vi "WaveformSimulatorFINAL.vi"(9 "Waveform Parameters":T1={"Frequency"=50.0, "Amplitude"=5.0, "Shape"=enum."Sine"}, 10 "Digitizing Parameters":T2={"Number of Samples"=100, "Sampling Frequency"=1000.0}) -> (2 "Waveform Output":cluster{"Time":dbl[], "Displacement":dbl[]}={"Time"=[0.0, 0.001, 0.002, 0.003, 0.004, 0.005, 0.006, 0.007, 0.008, 0.009000000000000001, 0.01, 0.011, 0.012, 0.013000000000000001, 0.014, 0.015, 0.016, 0.017, 0.018000000000000002, 0.019, 0.02, 0.021, 0.022, 0.023, 0.024, 0.025, 0.026000000000000002, 0.027, 0.028, 0.029, 0.03, 0.031, 0.032, 0.033, 0.034, 0.035, 0.036000000000000004, 0.037, 0.038, 0.039, 0.04, 0.041, 0.042, 0.043000000000000003, 0.044, 0.045, 0.046, 0.047, 0.048, 0.049, 0.05, 0.051000000000000004, 0.052000000000000005, 0.053, 0.054, 0.055, 0.056, 0.057, 0.058, 0.059000000000000004, 0.06, 0.061, 0.062, 0.063, 0.064, 0.065, 0.066, 0.067, 0.068, 0.069, 0.07, 0.07100000000000001, 0.07200000000000001, 0.073, 0.074, 0.075, 0.076, 0.077, 0.078, 0.079, 0.08, 0.081, 0.082, 0.083, 0.084, 0.085, 0.08600000000000001, 0.08700000000000001, 0.088, 0.089, 0.09, 0.091, 0.092, 0.093, 0.094, 0.095, 0.096, 0.097, 0.098, 0.099], "Displacement"=[0.0, 1.545084971874737, 2.938926261462366, 4.045084971874737, 4.755282581475767, 5.0, 4.755282581475767, 4.045084971874737, 2.9389262614623664, 1.5450849718747355, 6.123233995736766e-16, -1.5450849718747364, -2.938926261462367, -4.04508497187474, -4.755282581475767, -5.0, -4.755282581475768, -4.045084971874735, -2.938926261462363, -1.5450849718747381, -1.2246467991473533e-15, 1.54508497187474, 2.9389262614623646, 4.045084971874736, 4.755282581475769, 5.0, 4.7552825814757655, 4.045084971874738, 2.938926261462367, 1.545084971874739, 1.8369701987210296e-15, -1.5450849718747353, -2.938926261462364, -4.045084971874741, -4.75528258147577, -5.0, -4.755282581475766, -4.045084971874738, -2.9389262614623672, -1.5450849718747395, -2.4492935982947065e-15, 1.545084971874743, 2.938926261462371, 4.045084971874741, 4.755282581475767, 5.0, 4.755282581475769, 4.045084971874739, 2.9389262614623606, 1.5450849718747315, -5.82016719913287e-15, -1.5450849718747426, -2.9389262614623775, -4.045084971874741, -4.755282581475767, -5.0, -4.755282581475769, -4.045084971874734, -2.9389262614623686, -1.545084971874732, -3.673940397442059e-15, 1.545084971874742, 2.9389262614623624, 4.04508497187474, 4.755282581475766, 5.0, 4.755282581475764, 4.045084971874735, 2.9389262614623544, 1.5450849718747328, -1.3477304596986768e-14, -1.5450849718747415, -2.938926261462376, -4.045084971874729, -4.755282581475766, -5.0, -4.755282581475769, -4.045084971874735, -2.9389262614623695, -1.5450849718747333, -4.898587196589413e-15, 1.5450849718747408, 2.9389262614623757, 4.04508497187474, 4.755282581475772, 5.0, 4.755282581475764, 4.045084971874725, 2.9389262614623703, 1.5450849718747508, 5.5109105961630896e-15, -1.5450849718747404, -2.9389262614623615, -4.045084971874739, -4.755282581475766, -5.0, -4.755282581475765, -4.0450849718747355, -2.938926261462356, -1.5450849718747346]} {"Displacement" format="%.10g"; "Time" format="%.10g"})   [LabVIEW 2015]
uses:
  <vilib>/imath/engines/lvmath2/RunTimeEngine/Managers/WorkSpace/UID Generator.vi
  <vilib>/imath/engines/lvmath2/RunTimeEngine/RunTimeType/NIMS_RunTimeType_From StrictType (excl LVString).vi
  <instcachedir>/0/NIMS_RunTimeType_From StrictType (excl LVString)_EB1C38A9BC5048DA9ABDA8F781E54D21.lvgen/NIMS_RunTimeType_From StrictType (excl LVString)_EB1C38A9BC5048DA9ABDA8F781E54D21_000.vi
  <vilib>/imath/engines/lvmath2/RunTimeEngine/LocalVariableDefStatement/MC_LocalVariableDefStatement_Display.vi
  <vilib>/imath/engines/lvmath2/RunTimeEngine/RangeToken/NIMS_Range.vi
  <instcachedir>/0/NIMS_Range_D919CC09935940E88F755EC1C6F49AC1.lvgen/NIMS_Range_D919CC09935940E88F755EC1C6F49AC1_000.vi
  <vilib>/imathl/engines/lvmath/Functions/Error Handling/Create Error.vi
  <vilib>/imath/engines/lvmath2/RunTimeEngine/ArithmeticOperatorToken/NIMS_ArithmeticOperator_plus.vi
  <instcachedir>/0/NIMS_ArithmeticOperator_plus_A4F2756F5ADB4A0090E0DBD7C10701C8.lvgen/NIMS_ArithmeticOperator_plus_A4F2756F5ADB4A0090E0DBD7C10701C8_004.vi
  <vilib>/imath/engines/lvmath2/RunTimeEngine/BuiltInFunctions/gensignal/NIMS_gensignal(str,RS,RS,RS).vi
  <vilib>/imath/engines/lvmath2/RunTimeEngine/BuiltInFunctions/transpose/NIMS_transpose(GV).vi
  <instcachedir>/0/NIMS_transpose(GV)_1D76875BF542458FA31D2D0CC3E998C0.lvgen/NIMS_transpose(GV)_1D76875BF542458FA31D2D0CC3E998C0_000.vi
  <vilib>/imath/engines/lvmath2/RunTimeEngine/BuiltInFunctions/linramp/NIMS_linramp.vi
  <vilib>/imath/engines/lvmath2/RunTimeEngine/VariableToken/NIMS_VariableToken_CondDefined.vi
  <instcachedir>/0/NIMS_VariableToken_CondDefined_FE30D0A1BFB24F098D41DEBABFE96BE1.lvgen/NIMS_VariableToken_CondDefined_FE30D0A1BFB24F098D41DEBABFE96BE1_003.vi
  <vilib>/imath/engines/lvmath/Functions/Error Handling/MergeErrorsWrapper.vi
  <vilib>/imath/engines/lvmath2/RunTimeEngine/Managers/SymbolTable/Clear UID.vi
  <vilib>/imath/engines/lvmath2/RunTimeEngine/NodeEndStatement/NIMS_NodeEndStatement_Output.vi
  <instcachedir>/0/NIMS_NodeEndStatement_Output_53EC0D466D134D7ABD903AC30B43404B.lvgen/NIMS_NodeEndStatement_Output_53EC0D466D134D7ABD903AC30B43404B_005.vi
  <vilib>/imath/engines/lvmath2/RunTimeEngine/ErrorHandling/NIMS_Finalize Error.vi
  <vilib>/imath/engines/lvmath2/RunTimeEngine/Managers/SymbolTable/NIMS_WorkSpace.lvlib
panel:
  out "XY Graph":cluster{"t":dbl[], "x":dbl[]}(graph)={"t"=[0.0, 0.001, 0.002, 0.003, 0.004, 0.005, 0.006, 0.007, 0.008, 0.009000000000000001, 0.01, 0.011, 0.012, 0.013000000000000001, 0.014, 0.015, 0.016, 0.017, 0.018000000000000002, 0.019, 0.02, 0.021, 0.022, 0.023, 0.024, 0.025, 0.026000000000000002, 0.027, 0.028, 0.029, 0.03, 0.031, 0.032, 0.033, 0.034, 0.035, 0.036000000000000004, 0.037, 0.038, 0.039, 0.04, 0.041, 0.042, 0.043000000000000003, 0.044, 0.045, 0.046, 0.047, 0.048, 0.049, 0.05, 0.051000000000000004, 0.052000000000000005, 0.053, 0.054, 0.055, 0.056, 0.057, 0.058, 0.059000000000000004, 0.06, 0.061, 0.062, 0.063, 0.064, 0.065, 0.066, 0.067, 0.068, 0.069, 0.07, 0.07100000000000001, 0.07200000000000001, 0.073, 0.074, 0.075, 0.076, 0.077, 0.078, 0.079, 0.08, 0.081, 0.082, 0.083, 0.084, 0.085, 0.08600000000000001, 0.08700000000000001, 0.088, 0.089, 0.09, 0.091, 0.092, 0.093, 0.094, 0.095, 0.096, 0.097, 0.098, 0.099], "x"=[0.0, 1.545084971874737, 2.938926261462366, 4.045084971874737, 4.755282581475767, 5.0, 4.755282581475767, 4.045084971874737, 2.9389262614623664, 1.5450849718747355, 6.123233995736766e-16, -1.5450849718747364, -2.938926261462367, -4.04508497187474, -4.755282581475767, -5.0, -4.755282581475768, -4.045084971874735, -2.938926261462363, -1.5450849718747381, -1.2246467991473533e-15, 1.54508497187474, 2.9389262614623646, 4.045084971874736, 4.755282581475769, 5.0, 4.7552825814757655, 4.045084971874738, 2.938926261462367, 1.545084971874739, 1.8369701987210296e-15, -1.5450849718747353, -2.938926261462364, -4.045084971874741, -4.75528258147577, -5.0, -4.755282581475766, -4.045084971874738, -2.9389262614623672, -1.5450849718747395, -2.4492935982947065e-15, 1.545084971874743, 2.938926261462371, 4.045084971874741, 4.755282581475767, 5.0, 4.755282581475769, 4.045084971874739, 2.9389262614623606, 1.5450849718747315, -5.82016719913287e-15, -1.5450849718747426, -2.9389262614623775, -4.045084971874741, -4.755282581475767, -5.0, -4.755282581475769, -4.045084971874734, -2.9389262614623686, -1.545084971874732, -3.673940397442059e-15, 1.545084971874742, 2.9389262614623624, 4.04508497187474, 4.755282581475766, 5.0, 4.755282581475764, 4.045084971874735, 2.9389262614623544, 1.5450849718747328, -1.3477304596986768e-14, -1.5450849718747415, -2.938926261462376, -4.045084971874729, -4.755282581475766, -5.0, -4.755282581475769, -4.045084971874735, -2.9389262614623695, -1.5450849718747333, -4.898587196589413e-15, 1.5450849718747408, 2.9389262614623757, 4.04508497187474, 4.755282581475772, 5.0, 4.755282581475764, 4.045084971874725, 2.9389262614623703, 1.5450849718747508, 5.5109105961630896e-15, -1.5450849718747404, -2.9389262614623615, -4.045084971874739, -4.755282581475766, -5.0, -4.755282581475765, -4.0450849718747355, -2.938926261462356, -1.5450849718747346]}
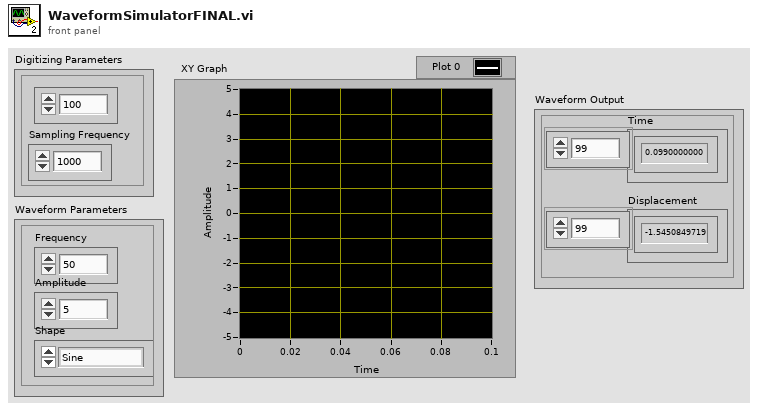
[diagram p1: front panel]
types:
  T1 = cluster{"Frequency":dbl, "Amplitude":dbl, "Shape":enum16{"Sine", "Cosine", "DC Level", "Square", "User-Defined"}}
  T2 = cluster{"Number of Samples":i32, "Sampling Frequency":dbl}
  T3 = enum16{"Sine", "Cosine", "DC Level", "Square", "User-Defined"}
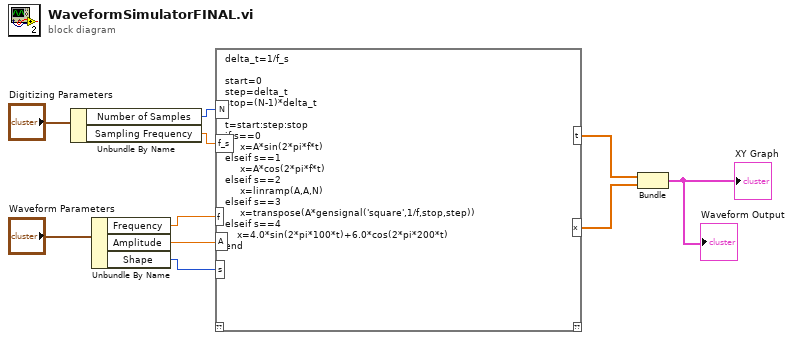
[diagram p0: block diagram]
diagram:
  n1 = Unbundle By Name("Digitizing Parameters") -> ("Number of Samples"=w6:i32, "Sampling Frequency"=w5:dbl)
  n2 = Unbundle By Name("Waveform Parameters") -> ("Frequency"=w4:dbl, "Amplitude"=w3:dbl, "Shape"=w2:T3)
  n3 = mathscript code="delta_t=1/f_s\n\nstart=0\nstep=delta_t\nstop=(N-1)*delta_t\n\nt=start:step:stop\nif s==0\n     x=A*sin(2*pi*f*t)\nelseif s==1\n     x=A*cos(2*pi*f*t)\nelseif s==2\n     x=linramp(A,A,N)\nelseif s==3\n     x=transpose(A*gensignal('square',1/f,stop,step))\nelseif s==4\n    x=4.0*sin(2*pi*100*t)+6.0*cos(2*pi*200*t)\nend"("N"=w6, "f_s"=w5, "f"=w4, "A"=w3, "s"=w2) -> ("t"=w10:dbl[], "x"=w9:dbl[])  [unwired: 1 in, 1 out]
  n4 = Bundle("t"=w10, "x"=w9) -> (→"XY Graph" →"Waveform Output":cluster{"t":dbl[], "x":dbl[]})  [unwired: 1 in]
